vi "Status Updated.vi"(8 "error in (no error)":errorcluster, 10 "Status":string) -> (0 "error out":errorcluster)   [LabVIEW 2021, in "Actuator Module.lvlib"]
doc: "Send the Status Updated event to any VI registered to listen to events from the owning library.\n_______\nCreated using Delacor User Event Scripter 1.0.0.6."
uses:
  Actuator Module.lvlib
  Status Updated Argument--cluster.ctl
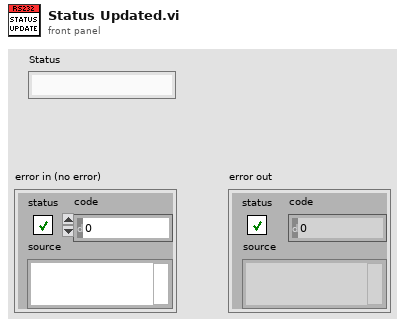
[diagram p1: front panel]
types:
  T1 = typedef "Actuator Module.lvlib/Status Updated Argument--cluster.ctl" = cluster{"Status":string}
  T2 = typedef "Actuator Module.lvlib/Broadcast Events--cluster.ctl" = cluster{"Status Updated":refnum<user-event>, "Actuator-display-Interface":refnum<user-event>}
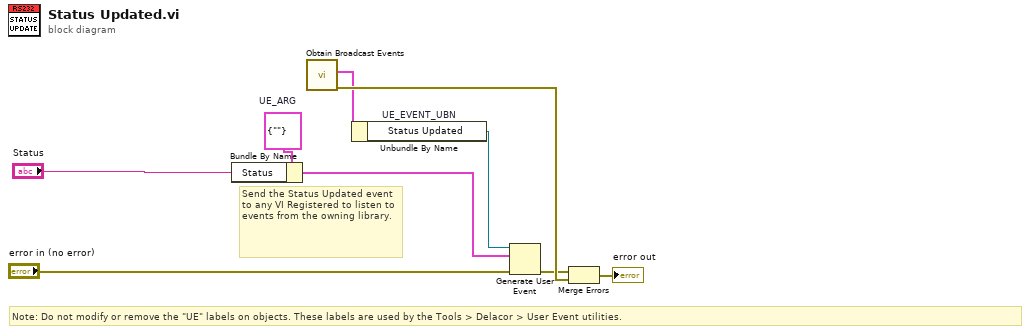
[diagram p0: block diagram]
diagram:
  w3 = T1 {"Status"=""}  # UE_ARG
  # "Note: Do not modify or remove the \"UE\" labels on objects. These labels are used by the Tools > Delacor > User Event utilities."
  # "Send the Status Updated event to any VI Registered to listen to events from the owning library."
  n1 = Bundle By Name(cluster=w3, "Status"="Status") -> (w2:T1)
  n2 = call "Obtain Broadcast Events.vi"() -> ("error out"=w7:errorcluster, "Actuator Module Broadcast Events"=w5:T2)  [unwired: 10 in]
  n3 = Unbundle By Name "UE_EVENT_UBN"(w5) -> ("Status Updated"=w4:refnum<user-event>)
  n4 = Generate User Event(user event=w4, event data cluster=w2, error in="error in (no error)") -> (error out=w6:errorcluster)  [unwired: 1 in, 1 out]
  n5 = Merge Errors(w6, w7) -> (→"error out":errorcluster)
